vi "Read datatype.vi"(8 "error in (no error)":errorcluster, 11 "JSON Boolean in":refnum<class "JSON Helper.lvclass">) -> (0 "error out":errorcluster, 2 "datatype":T1, 3 "JSON Boolean out":refnum<class "JSON Helper.lvclass">)   [LabVIEW 2016, in "JSON Boolean.lvclass"]
doc: "Returns the JSON Type of the given object. This may be used to determine if the value of a control of type JSON Null, JSON Literal or JSON Structured Type is an instance of a more specific type."
uses:
  JSON Boolean.lvclass
  JSON Types.ctl
  JSON Helper/JSON Helper.lvclass
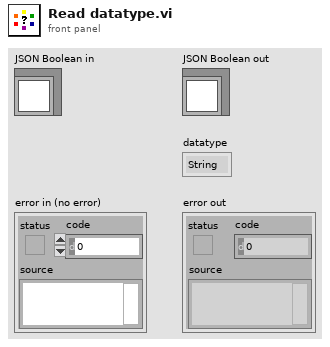
[diagram p1: front panel]
types:
  T1 = typedef "JSON Helper.lvclass/JSON Types.ctl" = enum16{"String", "Numeric", "Boolean", "NULL", "Object", "Array"}
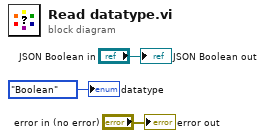
[diagram p0: block diagram]
diagram:
  "error out" <- "error in (no error)"
  "JSON Boolean out" <- "JSON Boolean in"
  "datatype" <- JSON_Types."Boolean" ("datatype")
